vi "Generate TF Process.vi"   [LabVIEW 2020]
uses:
  Process Generation/New Class Dialog/New Class Dialog.lvclass
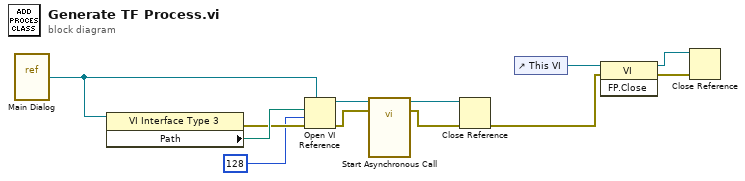
[diagram p0: block diagram]
diagram:
  n1 = vi-ref "Main Dialog.vi"() -> (w8:refnum<vi>)
  n2 = property class="VI Interface Type 3"(reference=w8) -> (error out=w6:errorcluster, "Path"=w7:path)  [unwired: 1 in, 1 out]
  n3 = Open VI Reference(type specifier VI Refnum (for type only)=w8, vi path=w7, options=128, error in (no error)=w6) -> (vi reference=w9:refnum<vi>, error out=w12:errorcluster)  [unwired: 2 in]
  n4 = call-by-ref "Start Asynchronous Call"(reference=w9, error in=w12) -> (reference out=w11:refnum<vi>, error out=w10:errorcluster)  [unwired: 12 in]
  n5 = Close Reference(reference=w11, error in (no error)=w10) -> (error out=w2:errorcluster)
  n6 = control-ref of="This VI"() -> (w1:refnum<vi>)
  n7 = invoke class="VI" method="FP.Close"(reference=w1, error in=w2) -> (reference out=w4:refnum<vi>, error out=w3:errorcluster)  [unwired: 1 in, 1 out]
  n8 = Close Reference(reference=w4, error in (no error)=w3) -> ()  [unwired: 1 out]
